vi "specu1a 1.0.0 Get Error Enum.vi"(4 "Error Code in":i16) -> (1 "Specu1a 1.0.0 Error code out":T1)   [LabVIEW 2019]
uses:
  Controls/specu1a 1.0.0 Error codes.ctl
panel:
  in  "Specu1a 1.0.0 Error codes":T1=enum."USBDEV_RW_EEP_ERROR"
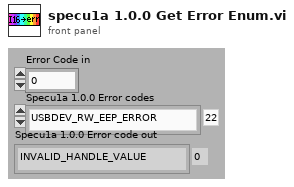
[diagram p1: front panel]
types:
  T1 = typedef "specu1a 1.0.0 Error codes.ctl" = enum16{"INVALID_HANDLE_VALUE", "USBDEV_SUCCESS", "USBDEV_INVALID_HANDLE", "USBDEV_UNSUCCESS", "USBDEV_INVALID_VALUE", "USBDEV_CHECK_NORMAL", "USBDEV_CHECK_INVALID", "USBDEV_CHECK_REMOVE", "USBDEV_CHECK_OTHER", "USBDEV_RESET_ERROR", "USBDEV_BULKSIZE_ERROR", "USBDEV_BULK_READ_ERROR", "USBDEV_BULK_NOT_UPDATED", "USBDEV_TIME_OVER_ERROR", "USBDEV_TIME_UNDER_ERROR", "USBDEV_TIME_SET_ERROR", "USBDEV_SET_GAIN_ERROR", "USBDEV_GET_TEMP_ERROR", "USBDEV_SET_TRIGGER_ERROR", "USBDEV_RW_EEP_ADDR_ERROR", "USBDEV_RW_EEP_SIZE_ERROR", "USBDEV_RW_EEP_OVER_ERROR", "USBDEV_RW_EEP_ERROR", "UNITID_PRODUCTID_CONFLICT", "UNKNOWN_ERROR"}
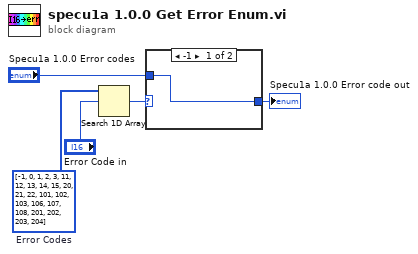
[diagram p0: block diagram]
diagram:
  w5 = i32[] [-1, 0, 1, 2, 3, 11, 12, 13, 14, 15, 20, 21, 22, 101, 102, 103, 106, 107, 108, 201, 202, 203, 204]  # Error Codes
  n1 = Search 1D Array(1D array=w5, element="Error Code in") -> (index of element=w1:i32)  [unwired: 1 in]
  n2 = case shown="-1" w1 {
    selector: w1 -> [_ w7]
    tunnel: "Specu1a 1.0.0 Error codes" -> [w6 _]
    tunnel: [w6 w7] -> w2
    frame -1 {
    }
    frame 0, Default {
    }
  }
  "Specu1a 1.0.0 Error code out" <- w2
